vi "State Variable FIlter.vi"(7 "initialize":bool, 8 "Fs":dbl, 9 "Q":dbl, 10 "Fc":dbl, 11 "x":dbl[](array[numeric]) format="%0.2f") -> (0 "Highpass":dbl[](array[numeric]) format="%0.2f", 1 "Bandpass":dbl[](array[numeric]) format="%0.2f", 2 "Lowpass":dbl[](array[numeric]) format="%0.2f")   [LabVIEW 2013]
doc: "Filters <B>x</B> using the cascade form of the IIR filter specified by the <B>IIR Filter Cluster</B>."
panel:
  # "Note: only stable for Fc < 1/6 Fs"
  # "Bessel = 0.57, Butterworth = 0.7"
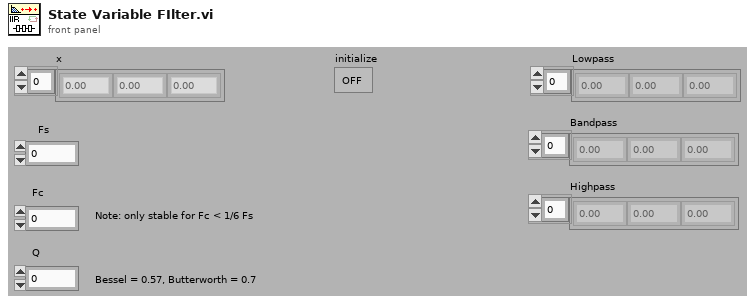
[diagram p1: front panel]
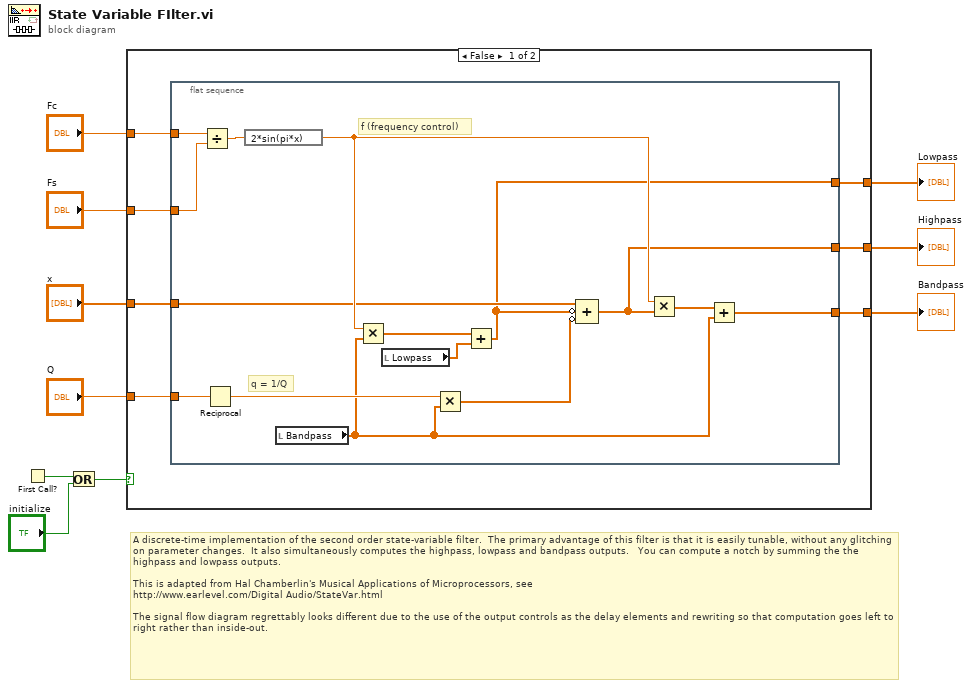
[diagram p0: block diagram]
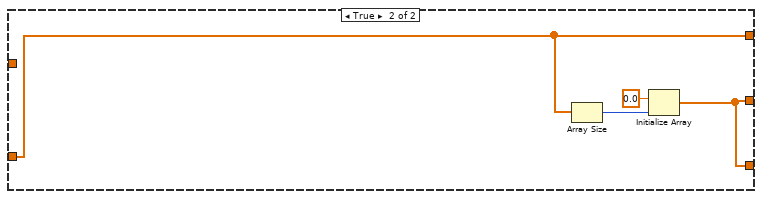
[diagram p2: hidden frame]
diagram:
  # "A discrete-time implementation of the second order state-variable filter.  The primary advantage of this filter is that it is easily tunable, without any glitching on parameter changes.  It also simultaneously computes the highpass, lowpass and bandpass outputs.   You can compute a notch by summing the the highpass and lowpass outputs.\n\nThis is adapted from Hal Chamberlin's Musical Applications of Microprocessors, see \nhttp://www.earlevel.com/Digital Audio/StateVar.html \n\nThe signal flow diagram regrettably looks different due to the use of the output controls as the delay elements and rewriting so that computation goes left to right rather than inside-out."
  n1 = First Call?() -> (First Call?: T/F=w10:bool)
  n2 = Or(x=w10, y="initialize") -> (x .or. y?=w1:bool)
  n3 = case shown="False" w1 {
    tunnel: "Q" -> [w17 _]
    tunnel: "Fc" -> [w16 _]
    tunnel: "Fs" -> [w15 _]
    tunnel: [w14 w33] -> w5
    tunnel: [w13 w36] -> w4
    tunnel: [w12 w33] -> w3
    tunnel: "x" -> [w11 w36]
    frame False {
      n4 = flat-sequence {
        tunnel: w17 -> [w32]
        tunnel: w16 -> [w31]
        tunnel: w15 -> [w30]
        tunnel: [w25] -> w14
        tunnel: [w18] -> w13
        tunnel: [w22] -> w12
        tunnel: w11 -> [w21]
        frame #0 {
          # "q = 1/Q"
          # "f (frequency control)"
          n5 = Divide(x=w31, y=w30) -> (x/y=w29:dbl)
          n6 = Reciprocal(x=w32) -> (1/x=w28:dbl)
          n7 = expression code="2*sin(pi*x)"(w29) -> (w24:dbl)
          n8 = local read "Bandpass"() -> (w19:dbl[])
          n9 = Multiply(x=w24, y=w19) -> (x*y=w23:dbl[])
          n10 = local read "Lowpass"() -> (w20:dbl[])
          n11 = Multiply(x=w28, y=w19) -> (x*y=w27:dbl[])
          n12 = Add(x=w23, y=w20) -> (x+y=w18:dbl[])
          n13 = Compound Arithmetic op=ADD(w21, invert w18, invert w27) -> (w22:dbl[])
          n14 = Multiply(x=w24, y=w22) -> (x*y=w26:dbl[])
          n15 = Add(x=w26, y=w19) -> (x+y=w25:dbl[])
        }
      }
    }
    frame True {
      n16 = Array Size(array=w36) -> (size(s)=w35:i32)
      n17 = Initialize Array(0.0 ("element"), w35) -> (w33:dbl[])
    }
  }
  "Lowpass" <- w4
  "Highpass" <- w3
  "Bandpass" <- w5
